vi "Main.vi"(11 "Module Admin":refnum<class "Delacor_lib_QMH_Module Admin.lvclass">) -> ()   [LabVIEW 2019, in "Filepath Editor.lvlib"]
doc: "This template is based off of the Queued Message Handler design pattern and the Queued Message Handler project template that ships with LabVIEW.\n\nThe main difference is that the queue is private to this module and communication between modules is performed via Broadcast and Request events.\n\nRequest events are wrapped in public API methods and are handled in the Event Handling Loop (EHL) of this VI. Any module can register for Broadcast events sent by this module. The EHL generates messages based on user interface actions.\n\nThe Message Handling Loop (MHL) processes messages generated by the EHL, or by other messages. The messages are string values, so new messages can be added easily to the Message Cases case structure in the MHL. Each message cluster can also provide an optional value for Message Data, which is a variant that can be converted to whatever message-specific data is required.\n_____\nBased on Delacor QMH Project Template 4.0.0.47.\n_____\nBased on DQMH Project Template 6.1.0.94."
uses:
  Filepath Editor.lvlib
  <vilib>/Delacor/Delacor QMH/Libraries/Module Admin_class/Delacor_lib_QMH_Module Admin.lvclass
  Module Data--cluster.ctl
  Settings--cluster.ctl
  Stop Argument--cluster.ctl
  <vilib>/Delacor/Delacor QMH/Libraries/Message Queue_class/Delacor_lib_QMH_Message Queue.lvclass/Delacor_lib_QMH_Message Queue.ctl
  <vilib>/Delacor/Delacor QMH/Libraries/Module Admin_class/Delacor_lib_QMH_Module Admin.lvclass/Delacor_lib_QMH_Module Admin.ctl
  <vilib>/Utility/miscctls.llb/LVPointTypeDef.ctl
  <vilib>/Delacor/Delacor QMH/Libraries/Message Queue_class/Delacor_lib_QMH_Enqueue Message (Single).vi
  <vilib>/Delacor/Delacor QMH/Libraries/Module Admin_class/Delacor_lib_QMH_Get External Launch.vi
  <vilib>/Utility/error.llb/Error Cluster From Error Code.vi
  <vilib>/ErrorRing/Error Ring.xnode
  <vilib>/Delacor/Delacor QMH/Libraries/Message Queue_class/Delacor_lib_QMH_Message Queue.lvclass
panel:
  in  "Dir?":bool=TRUE
  in  "TDMS Directory":path=path "C:/Users/Lorenzo/Desktop/25102023_PFQNM_VCAM1_THP1/25102023_PFQNM_VCAM1_THP1/Cell2"
  in  "Cancel":bool
  in  "OK":bool
  in  "TDMS filepath":path
  out "error out":errorcluster
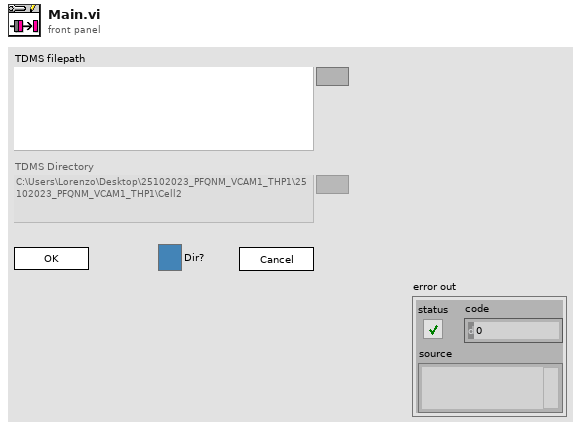
[diagram p1: front panel]
types:
  T1 = typedef "Filepath Editor.lvlib/Request Events--cluster.ctl" = cluster{"Stop Module":refnum<user-event>, "Show Panel":refnum<user-event>, "Hide Panel":refnum<user-event>, "Get Module Execution Status":refnum<user-event>, "Show Diagram":refnum<user-event>}
  T2 = typedef "Filepath Editor.lvlib/Module Data--cluster.ctl" = cluster{"Settings":T3}
  T3 = typedef "Filepath Editor.lvlib/Settings--cluster.ctl" = cluster{"TDMS Filepath":path, "TDMS Directory":path, "Dir?":bool}
  T4 = enum32{"invalid lock state", "Not Locked", "Locked (No Password)", "Password-protected"}
  T5 = typedef "Filepath Editor.lvlib/Stop Argument--cluster.ctl" = cluster{"Origin":string, "Exit via Stop Module Req?":bool, "Wait for Module to stop?":bool}
  T6 = typedef "LVPointTypeDef.ctl" = cluster{"Horizontal":i16, "Vertical":i16}
  T7 = enum32{"Invalid", "Standard", "Closed", "Hidden", "Minimized", "Maximized"}
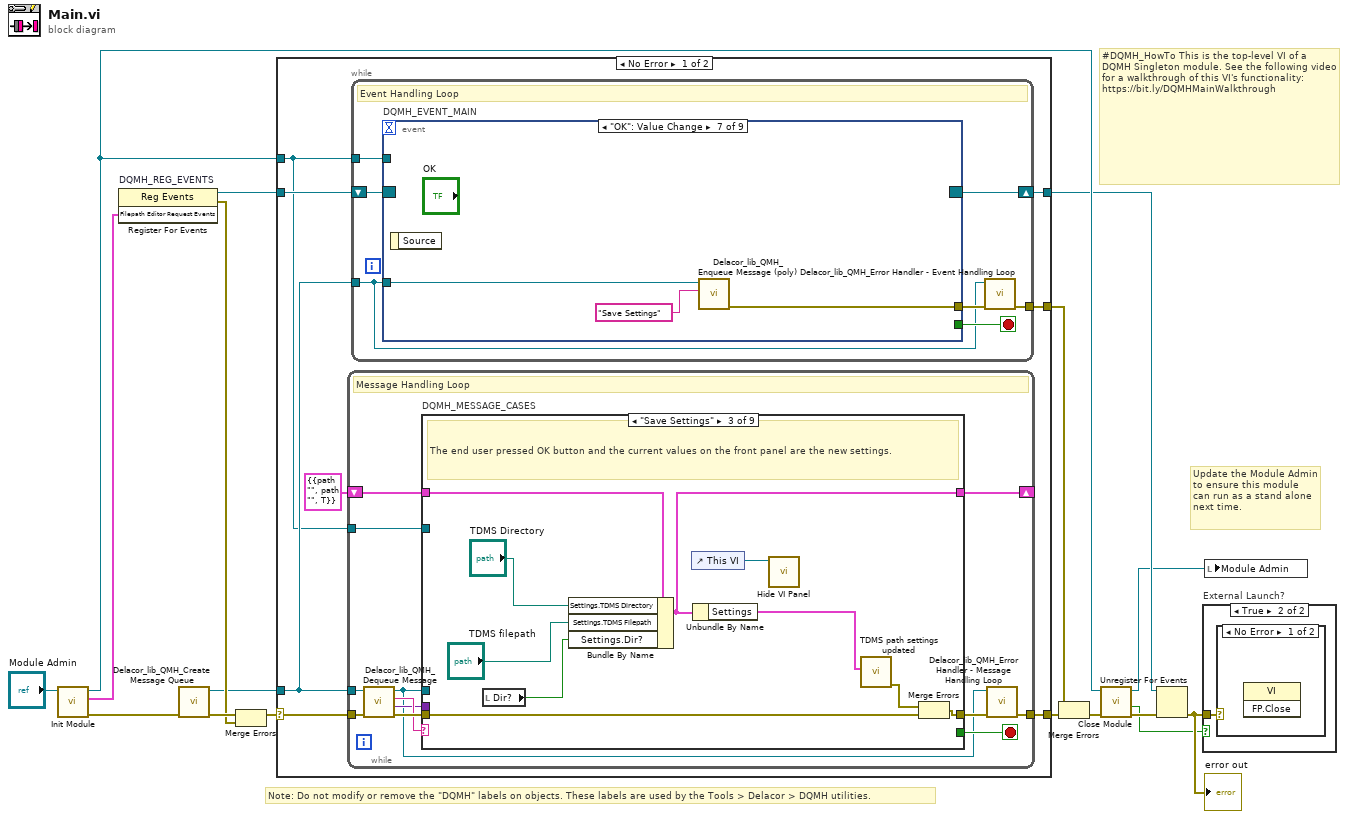
[diagram p0: block diagram]
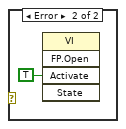
[diagram p3: hidden frame]
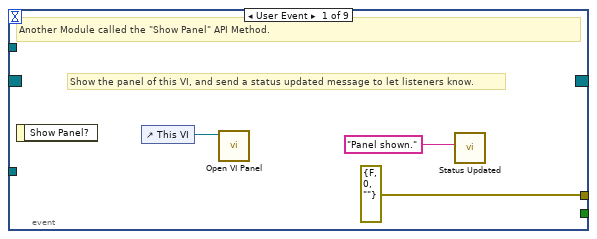
[diagram p4: hidden frame]
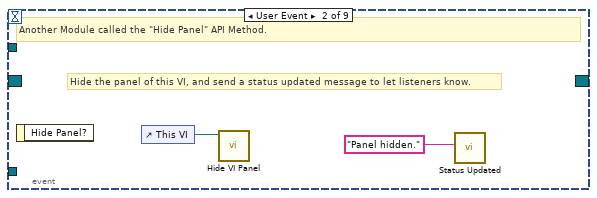
[diagram p5: hidden frame]
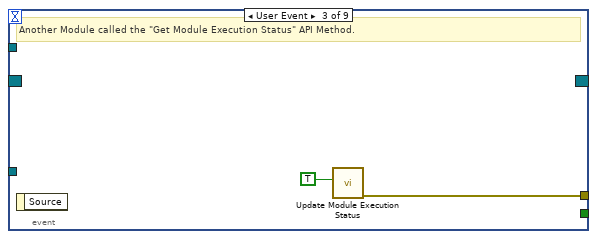
[diagram p6: hidden frame]
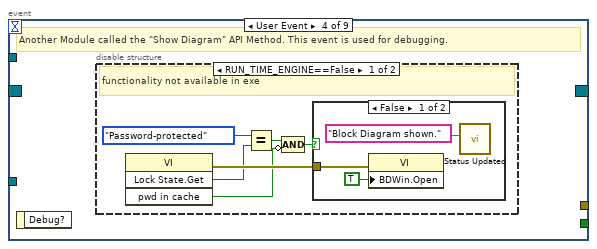
[diagram p7: hidden frame]
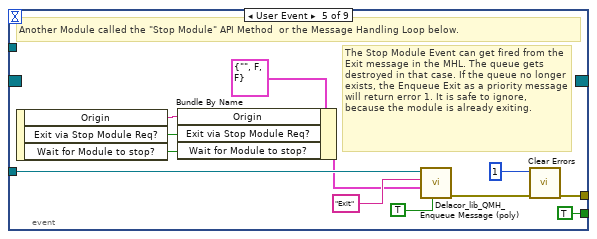
[diagram p10: hidden frame]
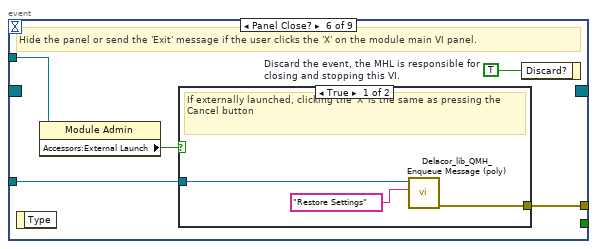
[diagram p11: hidden frame]
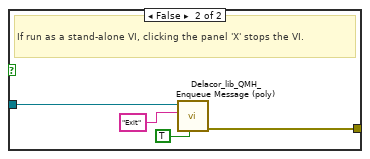
[diagram p12: hidden frame]
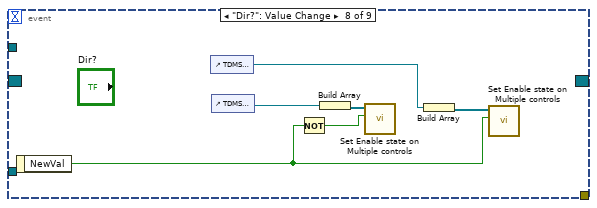
[diagram p13: hidden frame]
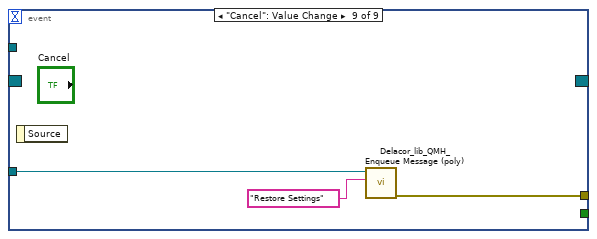
[diagram p14: hidden frame]
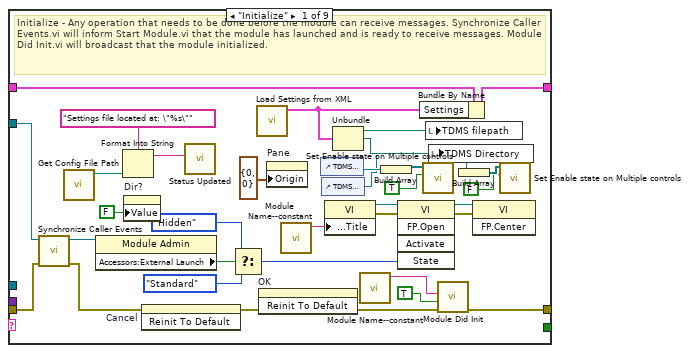
[diagram p15: hidden frame]
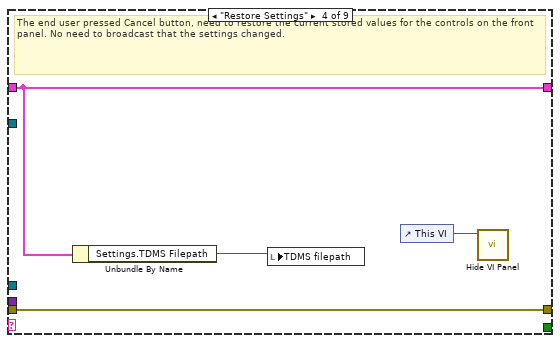
[diagram p17: hidden frame]
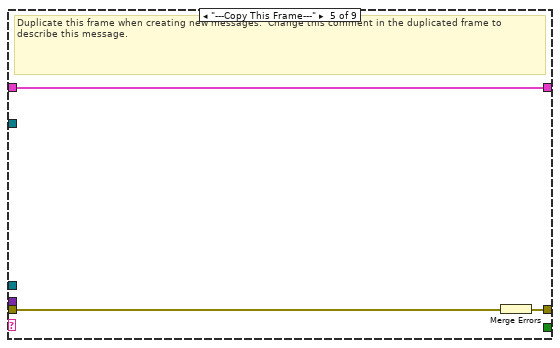
[diagram p18: hidden frame]
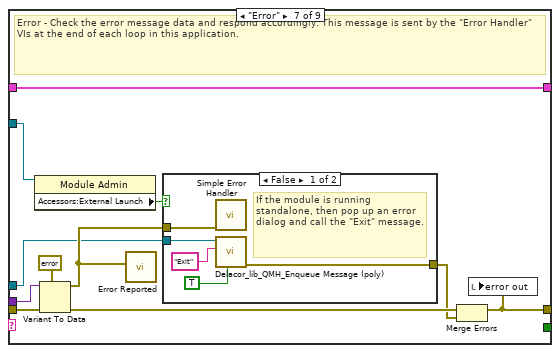
[diagram p20: hidden frame]
diagram:
  # "#DQMH_HowTo This is the top-level VI of a DQMH Singleton module. See the following video for a walkthrough of this VI's functionality: https://bit.ly/DQMHMainWalkthrough"
  # "Note: Do not modify or remove the \"DQMH\" labels on objects. These labels are used by the Tools > Delacor > DQMH utilities."
  # "Update the Module Admin to ensure this module can run as a stand alone next time."
  n1 = call "Init Module.vi"("Singleton Module Admin in"="Module Admin") -> ("error out"=w16:errorcluster, "Filepath Editor Request Events"=w5:T1, "Singleton Module Admin out"=w8:refnum<class "Delacor_lib_QMH_Module Admin.lvclass">)  [unwired: 8 in]
  n2 = register-events "DQMH_REG_EVENTS"(w5) -> (reference out=w6:refnum<event-registration>, error out=w9:errorcluster)  [unwired: 2 in]
  n3 = call <vilib>:"Delacor_lib_QMH_Create Message Queue.vi"("error in"=w16) -> ("error out"=w11:errorcluster, "Message Queue"=w4:refnum<class "Delacor_lib_QMH_Message Queue.lvclass">)  [unwired: 9 in]
  n4 = Merge Errors(w11, w9) -> (w10:errorcluster)
  n5 = case shown="No Error" w10 {
    selector: w10 -> [w23 w196]
    tunnel: [w25 w195] -> w17
    tunnel: [w22 w202] -> w7
    tunnel: w6 -> [w20 w202]
    tunnel: w4 -> [w19 w197]
    tunnel: [w24 _] -> w14
    tunnel: w8 -> [w18 w198]
    frame No Error {
      n6 = while {
        tunnel: w19 -> [w87]
        shift-right: [w91] -> _
        shift-left: T2 {"Settings"={"TDMS Filepath"=path "", "TDMS Directory"=path "", "Dir?"=TRUE}} ("Data Cluster") -> [w92]
        tunnel: w23 -> [w95]
        tunnel: [w93] -> w25
        tunnel: w18 -> [w85]
        stop <- w90 stop-if-true
        # "Message Handling Loop"
        n7 = call-dynamic "Delacor_lib_QMH_Dequeue Message.vi"("error in"=w95, "Message Queue in"=w87) -> ("error out"=w94:errorcluster, "Message Data"=w88:variant, "Message"=w89:string, "Message Queue out"=w86:refnum<class "Delacor_lib_QMH_Message Queue.lvclass">)  [unwired: 6 in]
        n8 = case "DQMH_MESSAGE_CASES" shown="\"Save Settings\"" w89 {
          selector: w89 -> [_ _ _ _ _ _ _ _ w182]
          tunnel: w86 -> [_ _ _ _ _ _ w152 w174 _]
          tunnel: w94 -> [w127 w130 w135 w144 w147 w149 w159 w180 w184]
          tunnel: [w125 w130 w136 w144 w146 w149 w155 w177 w185] -> w96
          tunnel: w92 -> [w116 w129 w140 w143 w145 w148 w154 w173 w183]
          tunnel: [w115 w129 w138 w143 w145 w148 w154 w173 w183] -> w91
          tunnel: [_ _ _ _ _ _ _ w172 _] -> w90
          tunnel: w88 -> [_ _ _ _ _ _ w153 w171 _]
          tunnel: w85 -> [w117 _ _ _ _ _ w151 w166 _]
          frame "Initialize" {
            # "Initialize - Any operation that needs to be done before the module can receive messages. Synchronize Caller Events.vi will inform Start Module.vi that the module has launched and is ready to receive messages. Module Did Init.vi will broadcast that the module initialized."
            n9 = call "Synchronize Caller Events.vi"("error in (no error)"=w127, "Singleton Module Admin in"=w117) -> ("error out"=w126:errorcluster, "Singleton Module Admin out"=w112:refnum<class "Delacor_lib_QMH_Module Admin.lvclass">)  [unwired: 8 in]
            n10 = call "Get Config File Path.vi"() -> ("XML File Path"=w109:path)  [unwired: 10 in, 1 out]
            n11 = property class="Module Admin"(reference=w112) -> ("Accessors:External Launch"=w121:bool)  [unwired: 1 in, 2 out]
            n12 = Format Into String(format string="Settings file located at: \"%s\"", w109) -> (resulting string=w108:string)  [unwired: 2 in, 1 out]
            n13 = property on="Dir?" class="Bool (strict)"("Value"=FALSE ("Dir?")) -> ()  [unwired: 2 in, 2 out]
            n14 = invoke on="Cancel" class="Bool" method="Reinit To Default"() -> ()  [unwired: 3 in, 3 out]
            n15 = call "Status Updated.vi"("Status"=w108) -> ()  [unwired: 10 in, 1 out]
            n16 = Select(t=T7."Hidden" ("State"), s=w121, f=T7."Standard" ("State")) -> (s? t:f=w118:T7)
            n17 = call "Load Settings from XML.vi"() -> ("Settings out"=w106:T3)  [unwired: 10 in, 1 out]
            n18 = invoke on="OK" class="Bool" method="Reinit To Default"() -> ()  [unwired: 3 in, 3 out]
            n19 = property on="Pane" class="Pane"("Origin"=T6 {"Horizontal"=0, "Vertical"=0}) -> ()  [unwired: 2 in, 2 out]
            n20 = call "Module Name--constant.vi"() -> ("Module Name"=w124:string)  [unwired: 11 in]
            n21 = control-ref of="TDMS filepath"() -> (w103:refnum<vi>)
            n22 = control-ref of="TDMS Directory"() -> (w102:refnum<vi>)
            n23 = property class="VI"("Front Panel.Title"=w124) -> (reference out=w123:refnum<vi>, error out=w110:errorcluster)  [unwired: 2 in]
            n24 = Unbundle(w106) -> ("TDMS Filepath"=w105:path, "TDMS Directory"=w104:path)  [unwired: 1 out]
            n25 = call "Module Name--constant.vi"() -> ("Module Name"=w113:string)  [unwired: 11 in]
            n26 = Build Array(w103) -> (w101:refnum<vi>[])
            n27 = invoke class="VI" method="FP.Open"(reference=w123, error in=w110, "State"=w118) -> (reference out=w122:refnum<vi>, error out=w128:errorcluster)  [unwired: 2 in, 3 out]
            n28 = Bundle By Name(cluster=w116, "Settings"=w106) -> (w115:T2)
            n29 = call "Set Enable state on Multiple controls.vi"("Enable?"=TRUE, "Controls"=w101) -> ()  [unwired: 10 in]
            n30 = local write "TDMS filepath"(w105) -> ()
            n31 = local write "TDMS Directory"(w104) -> ()
            n32 = call "Module Did Init.vi"("error in (no error)"=w126, "Initialized?"=TRUE, "Origin"=w113) -> ("error out"=w125:errorcluster)  [unwired: 8 in]
            n33 = Build Array(w102) -> (w100:refnum<vi>[])
            n34 = invoke class="VI" method="FP.Center"(reference=w122, error in=w128) -> ()  [unwired: 1 in, 3 out]
            n35 = call "Set Enable state on Multiple controls.vi"("Enable?"=FALSE, "Controls"=w100) -> ()  [unwired: 10 in]
          }
          frame "---Module Specific---" {
            # "Separator -- The following cases handle messages specific to this Module."
          }
          frame "Save Settings" {
            # "The end user pressed OK button and the current values on the front panel are the new settings."
            n36 = local read "Dir?"() -> (w131:bool)
            n37 = Bundle By Name(cluster=w140, "Settings.TDMS Directory"="TDMS Directory", "Settings.TDMS Filepath"="TDMS filepath", "Settings.Dir?"=w131) -> (w138:T2)
            n38 = control-ref of="This VI"() -> (w139:refnum<vi>)
            n39 = Unbundle By Name(w138) -> ("Settings"=w132:T3)
            n40 = call "Hide VI Panel.vi"("VI"=w139) -> ()  [unwired: 10 in, 1 out]
            n41 = call "TDMS path settings updated.vi"("Settings"=w132) -> ("error out"=w133:errorcluster)  [unwired: 10 in]
            n42 = Merge Errors(w133, w135) -> (w136:errorcluster)
          }
          frame "Restore Settings" {
            # "The end user pressed Cancel button, need to restore the current stored values for the controls on the front panel. No need to broadcast that the settings changed."
            n43 = Unbundle By Name(w143) -> ("Settings.TDMS Filepath"=w142:path)
            n44 = local write "TDMS filepath"(w142) -> ()
            n45 = control-ref of="This VI"() -> (w141:refnum<vi>)
            n46 = call "Hide VI Panel.vi"("VI"=w141) -> ()  [unwired: 10 in, 1 out]
          }
          frame "---Copy This Frame---" {
            # "Duplicate this frame when creating new messages.  Change this comment in the duplicated frame to describe this message."
            n47 = Merge Errors(w147) -> (w146:errorcluster)
          }
          frame "---Exit and Error Handling---" {
            # "Separator - The following cases handle errors and exit messages."
          }
          frame "Error" {
            # "Error - Check the error message data and respond accordingly. This message is sent by the \"Error Handler\" VIs at the end of each loop in this application."
            n48 = property class="Module Admin"(reference=w151) -> ("Accessors:External Launch"=w150:bool)  [unwired: 1 in, 2 out]
            n49 = Variant To Data(error in=w159, type=errorcluster {"status"=FALSE, "code"=0, "source"=""} ("error constant"), Variant=w153) -> (data=w160:errorcluster, error out=w157:errorcluster)
            n50 = call "Error Reported.vi"("Error"=w160) -> ()  [unwired: 10 in, 1 out]
            n51 = case shown="False" w150 {
              tunnel: [w165 _] -> w156
              tunnel: w152 -> [w163 _]
              tunnel: w160 -> [w164 _]
              frame False {
                # "If the module is running standalone, then pop up an error dialog and call the \"Exit\" message."
                n52 = call <vilib>:"Simple Error Handler.vi"("error in (no error)"=w164) -> ()  [unwired: 4 in, 5 out]
                n53 = call-poly <vilib>:"Delacor_lib_QMH_Enqueue Message (poly).vi"("Priority Message? (F)"=TRUE, "Message"="Exit", "Message Queue in"=w163) -> ("error out"=w165:errorcluster)  [unwired: 7 in, 1 out]
              }
              frame True {
                # "If the module was launched externally, calling the Error Reported broadcast VI is the only action performed by the \"Error\" message. The module's caller can then process the error appropriately."
              }
            }
            n54 = Merge Errors(w157, w156) -> (w155:errorcluster)
            n55 = local write "error out"(w155) -> ()
          }
          frame "Exit" {
            w170 = 91  # 91: not all Exit messages will have an argument
            w172 = TRUE  # Stop the VI
            # "Release the message queue reference"
            # "Exit - Exit the application."
            n56 = Variant To Data(error in=w180, type=T5 {"Origin"="", "Exit via Stop Module Req?"=FALSE, "Wait for Module to stop?"=FALSE} ("Stop Argument"), Variant=w171) -> (data=w168:T5, error out=w176:errorcluster)
            n57 = call <vilib>:"Clear Errors.vi"("error in (no error)"=w176, "specific error code to clear (0: all)"=w170) -> ("error out"=w179:errorcluster)  [unwired: 4 in, 1 out]
            n58 = control-ref of="This VI"() -> (w167:refnum<vi>)
            n59 = call-dynamic "Delacor_lib_QMH_Release Message Queue.vi"("error in"=w179, "Message Queue"=w174) -> ("error out"=w178:errorcluster)  [unwired: 9 in]
            n60 = call "Handle Exit.vi"("Stop Argument"=w168, "Admin in"=w166, "VI reference"=w167) -> ("error out"=w175:errorcluster)  [unwired: 7 in, 1 out]
            n61 = Merge Errors(w178, w175) -> (w177:errorcluster)
          }
          frame Default {
            # "'Default' case only runs if there is a message that isn't defined in any of the other cases.  Output a programming error."
            n62 = call "Module Name--constant.vi"() -> ("Module Name"=w181:string)  [unwired: 11 in]
            n63 = xnode "Error Ring"("parameter 0"=w182, "parameter 1"=w181) -> ("error out"=w186:errorcluster)
            n64 = Merge Errors(w184, w186) -> (w185:errorcluster)
          }
        }
        n65 = call-dynamic "Delacor_lib_QMH_Error Handler - Message Handling Loop.vi"("error in"=w96, "Message Queue in"=w86) -> ("dup error in"=w93:errorcluster)  [unwired: 8 in, 1 out]
      }
      n66 = while {
        tunnel: w19 -> [w26]
        shift-right: [w29] -> w22
        shift-left: w20 -> [w30]
        tunnel: [w31] -> w24
        tunnel: w18 -> [w27]
        stop <- w28 stop-if-true
        # "Event Handling Loop"
        n67 = event "DQMH_EVENT_MAIN" shown="[6] \"OK\": Value Change" {
          selector: w30 -> [_ _ _ _ _ _ _ _ _]
          dyn-events: [_ _ _ _ _ _ _ _ _] -> w29
          timeout: _ -> [_ _ _ _ _ _ _ _ _]
          tunnel: [_ _ _ _ TRUE ("Discard?") _ _ _ _] -> w28
          tunnel: w26 -> [_ _ _ _ w56 w63 w73 _ w83]
          tunnel: [errorcluster {"status"=FALSE, "code"=0, "source"=""} ("error out") _ w39 _ w59 w65 w74 _ w82] -> w32
          tunnel: w27 -> [_ _ _ _ _ w62 _ _ _]
          event User Event {
            # "Show the panel of this VI, and send a status updated message to let listeners know."
            # "Another Module called the \"Show Panel\" API Method."
            n68 = event-data() -> ()  [unwired: 1 in, 1 out]
            n69 = control-ref of="This VI"() -> (w35:refnum<vi>)
            n70 = call "Open VI Panel.vi"("VI"=w35) -> ()  [unwired: 10 in, 1 out]
            n71 = call "Status Updated.vi"("Status"="Panel shown." ("format string")) -> ()  [unwired: 10 in, 1 out]
          }
          event User Event {
            # "Hide the panel of this VI, and send a status updated message to let listeners know."
            # "Another Module called the \"Hide Panel\" API Method."
            n72 = event-data() -> ()  [unwired: 1 in, 1 out]
            n73 = control-ref of="This VI"() -> (w37:refnum<vi>)
            n74 = call "Hide VI Panel.vi"("VI"=w37) -> ()  [unwired: 10 in, 1 out]
            n75 = call "Status Updated.vi"("Status"="Panel hidden." ("format string")) -> ()  [unwired: 10 in, 1 out]
          }
          event User Event {
            # "Another Module called the \"Get Module Execution Status\" API Method."
            n76 = event-data() -> ()  [unwired: 1 in, 1 out]
            n77 = call "Update Module Execution Status.vi"("Running?"=TRUE) -> ("error out"=w39:errorcluster)  [unwired: 10 in]
          }
          event User Event {
            # "Another Module called the \"Show Diagram\" API Method. This event is used for debugging."
            n78 = event-data() -> ()  [unwired: 1 in, 1 out]
            n79 = disable-structure shown="RUN_TIME_ENGINE==False" {
              frame condition #0 (active) {
                # "functionality not available in exe"
                n80 = invoke class="VI" method="Lock State.Get"() -> (error out=w45:errorcluster, "Get Lock State"=w44:T4, "pwd in cache"=w41:bool)  [unwired: 4 in, 1 out]
                n81 = Equal?(x=T4."Password-protected", y=w44) -> (x = y?=w42:bool)
                n82 = Compound Arithmetic op=AND(w42, invert w41) -> (w40:bool)
                n83 = case shown="False" w40 {
                  tunnel: w45 -> [w48 _]
                  frame False {
                    n84 = property class="VI"(error in=w48, "BDWin.Open"=TRUE ("Block Diagram Window:Open")) -> ()  [unwired: 1 in, 2 out]
                    n85 = call "Status Updated.vi"("Status"="Block Diagram shown." ("format string")) -> ()  [unwired: 10 in, 1 out]
                  }
                  frame True {
                    # "Password-protected VI, and the password is not in the cache. Do not show the diagram."
                  }
                }
              }
              frame condition #1 {
              }
            }
          }
          event User Event {
            # "The Stop Module Event can get fired from the Exit message in the MHL. The queue gets destroyed in that case. If the queue no longer exists, the Enqueue Exit as a priority message will return error 1. It is safe to ignore, because the module is already exiting."
            # "Another Module called the \"Stop Module\" API Method  or the Message Handling Loop below."
            n86 = event-data() -> ("Origin"=w49:string, "Exit via Stop Module Req?"=w52:bool, "Wait for Module to stop?"=w51:bool)  [unwired: 1 in]
            n87 = Bundle By Name(cluster=T5 {"Origin"="", "Exit via Stop Module Req?"=FALSE, "Wait for Module to stop?"=FALSE} ("Stop Argument"), "Origin"=w49, "Exit via Stop Module Req?"=w52, "Wait for Module to stop?"=w51) -> (w50:T5)
            n88 = call-poly <vilib>:"Delacor_lib_QMH_Enqueue Message (poly).vi"("Priority Message? (F)"=TRUE, "Message Data"=w50, "Message"="Exit", "Message Queue in"=w56) -> ("error out"=w60:errorcluster)  [unwired: 6 in, 1 out]
            n89 = call <vilib>:"Clear Errors.vi"("error in (no error)"=w60, "specific error code to clear (0: all)"=1) -> ("error out"=w59:errorcluster)  [unwired: 4 in, 1 out]
          }
          event Panel Close? {
            w64 = TRUE  # Discard the event, the MHL is responsible for closing and stopping this VI.
            # "Hide the panel or send the 'Exit' message if the user clicks the 'X' on the module main VI panel."
            n90 = event-data() -> ()  [unwired: 1 in, 1 out]
            n91 = property class="Module Admin"(reference=w62) -> ("Accessors:External Launch"=w61:bool)  [unwired: 1 in, 2 out]
            n92 = case shown="True" w61 {
              tunnel: w63 -> [w67 w71]
              tunnel: [w66 w72] -> w65
              frame True {
                # "If externally launched, clicking the 'X' is the same as pressing the Cancel button"
                n93 = call-poly <vilib>:"Delacor_lib_QMH_Enqueue Message (poly).vi"("Message"="Restore Settings", "Message Queue in"=w67) -> ("error out"=w66:errorcluster)  [unwired: 8 in, 1 out]
              }
              frame False {
                # "If run as a stand-alone VI, clicking the panel 'X' stops the VI."
                n94 = call-poly <vilib>:"Delacor_lib_QMH_Enqueue Message (poly).vi"("Priority Message? (F)"=TRUE, "Message"="Exit", "Message Queue in"=w71) -> ("error out"=w72:errorcluster)  [unwired: 7 in, 1 out]
              }
            }
            n95 = event-data("Discard?"=w64) -> ()  [unwired: 1 in, 1 out]
          }
          event "OK": Value Change {
            n96 = event-data() -> ()  [unwired: 1 in, 1 out]
            n97 = call-poly <vilib>:"Delacor_lib_QMH_Enqueue Message (poly).vi"("Message"="Save Settings", "Message Queue in"=w73) -> ("error out"=w74:errorcluster)  [unwired: 8 in, 1 out]
          }
          event "Dir?": Value Change {
            n98 = event-data() -> ("NewVal"=w76:bool)  [unwired: 1 in]
            n99 = control-ref of="TDMS Directory"() -> (w81:refnum<vi>)
            n100 = control-ref of="TDMS filepath"() -> (w79:refnum<vi>)
            n101 = Not(x=w76) -> (.not. x?=w77:bool)
            n102 = Build Array(w79) -> (w78:refnum<vi>[])
            n103 = call "Set Enable state on Multiple controls.vi"("Enable?"=w77, "Controls"=w78) -> ()  [unwired: 10 in]
            n104 = Build Array(w81) -> (w80:refnum<vi>[])
            n105 = call "Set Enable state on Multiple controls.vi"("Enable?"=w76, "Controls"=w80) -> ()  [unwired: 10 in]
          }
          event "Cancel": Value Change {
            n106 = event-data() -> ()  [unwired: 1 in, 1 out]
            n107 = call-poly <vilib>:"Delacor_lib_QMH_Enqueue Message (poly).vi"("Message"="Restore Settings", "Message Queue in"=w83) -> ("error out"=w82:errorcluster)  [unwired: 8 in, 1 out]
          }
        }
        n108 = call-dynamic "Delacor_lib_QMH_Error Handler - Event Handling Loop.vi"("error in"=w32, "Message Queue in"=w26) -> ("dup error in"=w31:errorcluster)  [unwired: 8 in, 1 out]
      }
    }
    frame Error {
      # "Synchronize Caller Events.vi will inform Start Module.vi that the module has launched and will let the code calling Start Module.vi register for broadcasts and would permit the caller receive the broadcast that an error occurred at launch time."
      n109 = call "Synchronize Caller Events.vi"("Singleton Module Admin in"=w198) -> ("error out"=w203:errorcluster)  [unwired: 9 in, 1 out]
      n110 = call-dynamic "Delacor_lib_QMH_Release Message Queue.vi"("error in"=w196, "Message Queue"=w197) -> ("error out"=w195:errorcluster)  [unwired: 9 in]
      n111 = call "Module Name--constant.vi"() -> ("Module Name"=w201:string)  [unwired: 11 in]
      n112 = Format Into String(format string="An error occurred during initialization. %s is no longer running.", w201) -> (resulting string=w199:string)  [unwired: 2 in, 1 out]
      n113 = Merge Errors(w195, w203) -> (w204:errorcluster)
      n114 = call "Error Reported.vi"("Additional Information"=w199, "Error"=w204) -> ()  [unwired: 9 in, 1 out]
    }
  }
  n115 = Merge Errors(w14, w17) -> (w13:errorcluster)
  n116 = call "Close Module.vi"("error in (no error)"=w13, "Module Admin in"=w8) -> ("error out"=w15:errorcluster, "External Launch"=w1:bool, "Module Admin out"=w2:refnum<class "Delacor_lib_QMH_Module Admin.lvclass">)  [unwired: 7 in]
  n117 = Unregister For Events(event registration refnum=w7, error in=w15) -> (error out=w12:errorcluster)
  "error out" <- w12
  n118 = case "External Launch?" shown="True" w1 {
    tunnel: w12 -> [_ w205]
    frame False {
    }
    frame True {
      n119 = case shown="No Error" w205 {
        frame No Error {
          n120 = invoke class="VI" method="FP.Close"() -> ()  [unwired: 3 in, 3 out]
        }
        frame Error {
          n121 = invoke class="VI" method="FP.Open"("Activate"=TRUE ("Activate?")) -> ()  [unwired: 4 in, 5 out]
        }
      }
    }
  }
  n122 = local write "Module Admin"(w2) -> ()
